vi "BNT_SLTag Subscription.vi"() -> ()   [LabVIEW 2019]
doc: "Synchronously sends messages to and receives messages from the Client VI using the Skyline Message API."
uses:
  <vilib>/Skyline/Message/AMQP/async/Open (Async).vi
  <vilib>/Skyline/Message/AMQP/NI Skyline Message AMQP (Async).lvclass
  <vilib>/Skyline/Message/NI Skyline Message.lvclass
panel:
  out "Received Message":string
  # "Overview: Demonstrates the use of the SystemLink Message functions to asynchronously send and receive messages\nRequirements: LabVIEW Base Development System\n                            SystemLink API\nInstructions:\n1. Ensure the server is running locally or the system running this VI is managed by the server.\n2. Run the VI either on the host or on a Real-Time target.\n3. Open & run the Host VI if it isn't running already.\n4. Watch the Received Message field to watch for messages received from the Host."
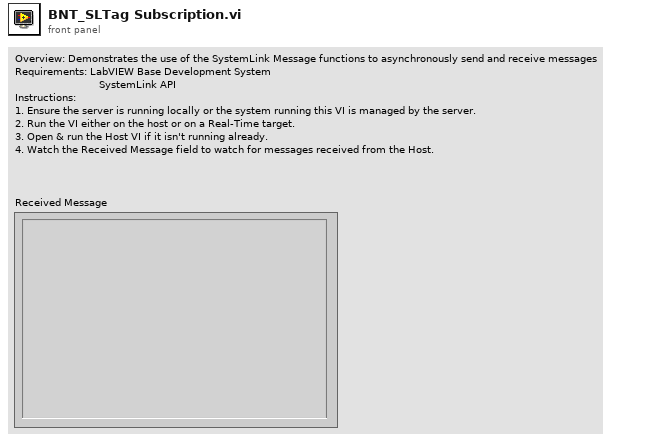
[diagram p1: front panel]
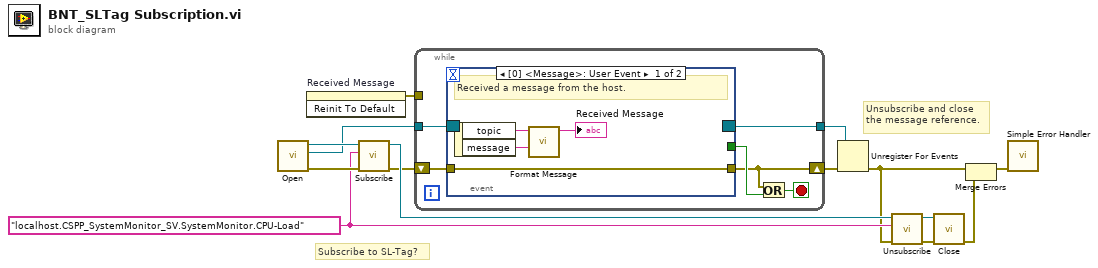
[diagram p0: block diagram]
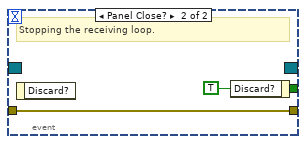
[diagram p2: hidden frame]
diagram:
  w7 = "localhost.CSPP_SystemMonitor_SV.SystemMonitor.CPU-Load" ("topic")
  # "Subscribe to SL-Tag?"
  # "Unsubscribe and close the message reference."
  n1 = call-poly <vilib>:"Open.vi"() -> ("error out"=w12:errorcluster, "event registration refnum"=w3:refnum<event-registration>, "message session"=w13:refnum<class "NI Skyline Message AMQP (Async).lvclass">)  [unwired: 9 in]
  n2 = invoke on="Received Message" class="Str" method="Reinit To Default"() -> (error out=w11:errorcluster)  [unwired: 3 in, 2 out]
  n3 = call-dynamic "Subscribe.vi"("error in (no error)"=w12, "topic"=w7, "message session in"=w13) -> ("error out"=w4:errorcluster, "message session out"=w5:refnum<class "NI Skyline Message AMQP (Async).lvclass">)  [unwired: 7 in]
  n4 = while {
    tunnel: [w18] -> w1
    shift-right: [w16] -> w14
    shift-left: w4 -> [w20]
    tunnel: w11 -> [_]
    tunnel: w3 -> [w15]
    stop <- w17 stop-if-true
    n5 = event shown="[0] <Message>: User Event" {
      selector: w15 -> [_ _]
      dyn-events: [_ _] -> w18
      timeout: _ -> [_ _]
      tunnel: w20 -> [w21 w26]
      tunnel: [_ w25] -> w19
      tunnel: [w21 w26] -> w16
      event User Event {
        # "Received a message from the host."
        n6 = event-data() -> ("topic"=w24:string, "message"=w22:string)  [unwired: 1 in]
        n7 = call "Format Message.vi"("message"=w22, "topic"=w24) -> ("formatted"=→"Received Message":string)  [unwired: 9 in]
      }
      event Panel Close? {
        w25 = TRUE ("Discard?")
        # "Stopping the receiving loop."
        n8 = event-data() -> ()  [unwired: 1 in, 1 out]
        n9 = event-data("Discard?"=w25) -> ()  [unwired: 1 in, 1 out]
      }
    }
    n10 = Or(x=w16, y=w19) -> (x .or. y?=w17:bool)
  }
  n11 = Unregister For Events(event registration refnum=w1, error in=w14) -> (error out=w2:errorcluster)
  n12 = call-dynamic "Unsubscribe.vi"("error in (no error)"=w2, "topic"=w7, "message session in"=w5) -> ("error out"=w10:errorcluster, "message session out"=w9:refnum<class "NI Skyline Message AMQP (Async).lvclass">)  [unwired: 7 in]
  n13 = call-dynamic "Close.vi"("error in (no error)"=w10, "message session"=w9) -> ("error out"=w6:errorcluster)  [unwired: 9 in]
  n14 = Merge Errors(w2, w6) -> (w8:errorcluster)
  n15 = call <vilib>:"Simple Error Handler.vi"("error in (no error)"=w8) -> ()  [unwired: 4 in, 5 out]
